vi "GV line clock start.vi"() -> ()   [LabVIEW 2017]
panel:
  out "Line clock start":bool
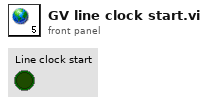
[diagram p1: front panel]
diagram:
